vi "NumericArrayToStringArray.vi"(11 "Array":dbl[][](array[numeric])) -> (3 "Array 2":string[][](array[string]))   [LabVIEW 2013]
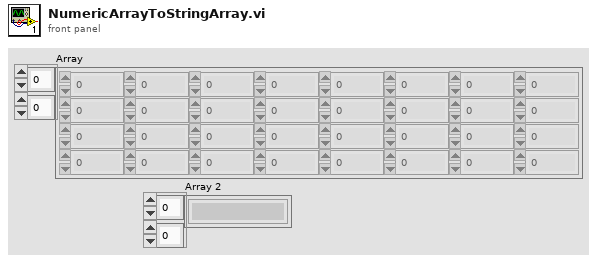
[diagram p1: front panel]
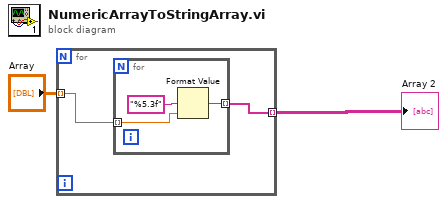
[diagram p0: block diagram]
diagram:
  n1 = for {
    tunnel: "Array" -> [w3] mode=indexing
    tunnel: [w4] -> w1 mode=indexing
    n2 = for {
      tunnel: [w7] -> w4 mode=indexing
      tunnel: w3 -> [w5] mode=indexing
      n3 = Format Value(format string="%5.3f", value (0)=w5) -> (output string=w7:string)  [unwired: 1 in]
    }
  }
  "Array 2" <- w1
